vi "IMAQController.SaveImages.vi"(0 "Scan Variables":T1, 1 "Save path in":path, 2 "Scan running?":bool, 3 "Acquisition Mode":T2(ring), 4 "serviceName":string, 5 "error in (no error)":errorcluster) -> (14 "Save path out Scan folder":path, 15 "Save path out Rainbow":path, 16 "Save path out Original":path, 17 "Save path out Horizontal":path, 18 "Save path out Verical":path, 19 "error out":errorcluster)   [LabVIEW 2014, in "IMAQController.lvlib"]
uses:
  IMAQController.lvlib
  CSlibraries-extern/DimLVEvent/LVDimInterface/LVDimInterface.lvlib
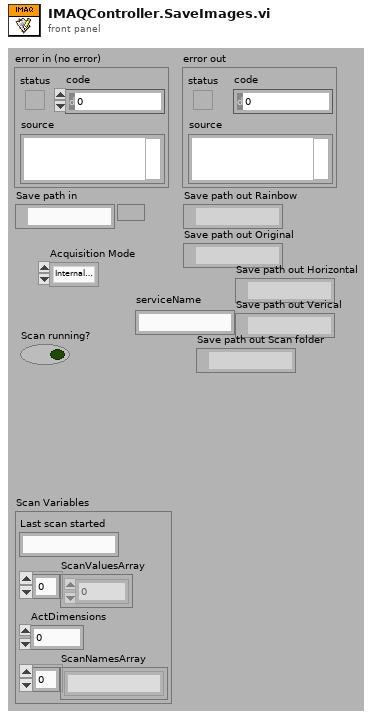
[diagram p1: front panel]
types:
  T1 = cluster{"Last scan started":string, "ScanValuesArray":dbl[], "ActDimensions":i16, "ScanNamesArray":string[]}
  T2 = enum32{"Internal Trigger", "Scan", "free Running", "External Trigger"}
  T3 = typedef "LVDateTimeRec.ctl" = cluster{"fractional second":dbl, "second":i32, "minute":i32, "hour":i32, "day of month":i32, "month":i32, "year":i32, "day of week":i32, "day of year":i32, "DST":i32}
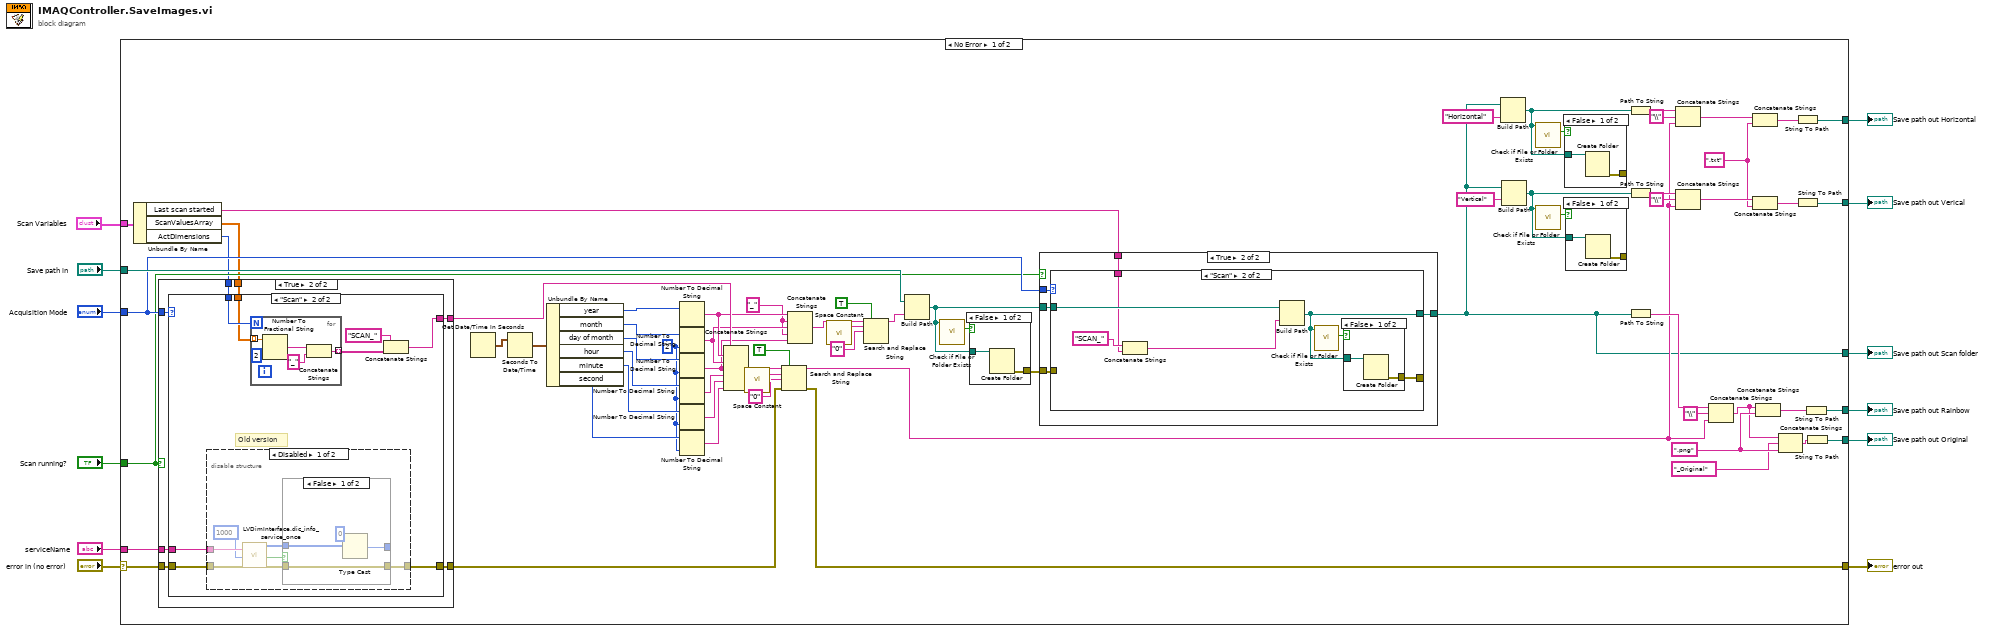
[diagram p0: block diagram]
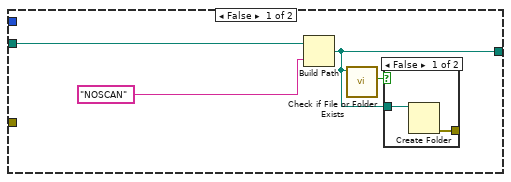
[diagram p2: hidden frame]
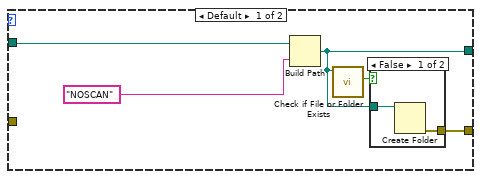
[diagram p4: hidden frame]
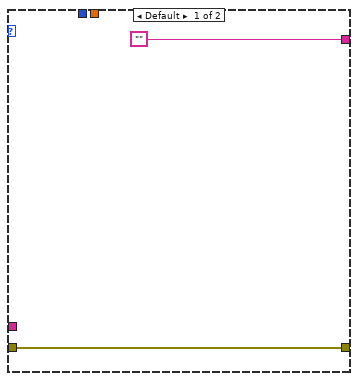
[diagram p8: hidden frame]
diagram:
  n1 = case shown="No Error" "error in (no error)" {
    selector: "error in (no error)" -> [w62 w150]
    tunnel: [w68 w150] -> w12
    tunnel: "Save path in" -> [w49 _]
    tunnel: [w64 _] -> w10
    tunnel: "Acquisition Mode" -> [w47 _]
    tunnel: "serviceName" -> [w60 _]
    tunnel: [w58 _] -> w7
    tunnel: [w21 _] -> w5
    tunnel: [w20 _] -> w4
    tunnel: "Scan Variables" -> [w19 _]
    tunnel: [w18 _] -> w3
    tunnel: "Scan running?" -> [w16 _]
    frame No Error {
      w24 = ".txt" ("string")
      w51 = "_"
      w56 = ".png" ("string")
      w70 = i16 2 ("width (-)")
      n2 = Unbundle By Name(w19) -> ("Last scan started"=w15:string, "ScanValuesArray"=w13:dbl[], "ActDimensions"=w14:i16)
      n3 = case shown="True" w16 {
        tunnel: [_ w115] -> w63
        tunnel: w62 -> [w108 w114]
        tunnel: [w108 w113] -> w61
        tunnel: w60 -> [_ w112]
        tunnel: w47 -> [_ w111]
        tunnel: w14 -> [_ w110]
        tunnel: w13 -> [_ w109]
        frame False {
        }
        frame True {
          n4 = case shown="\"Scan\"" w111 {
            tunnel: ["" w118] -> w115
            tunnel: w114 -> [w116 w125]
            tunnel: [w116 w123] -> w113
            tunnel: w112 -> [_ w124]
            tunnel: w110 -> [_ w122]
            tunnel: w109 -> [_ w121]
            frame Default {
            }
            frame "Scan" {
              # "Old version"
              n5 = disable-structure shown="Disabled" {
                disable-tunnel: w125 -> [w132 w138]
                disable-tunnel: w124 -> [w131 _]
                disable-tunnel: [w126 w138] -> w123
                frame Disabled {
                  n6 = call "LVDimInterface.dic_info_service_once.vi"("serviceName"=w131, "timeout [ms]"=u32 1000, "error in (no error)"=w132) -> ("data"=w129:i8[], "timed out?"=w127:bool, "error out"=w128:errorcluster)  [unwired: 13 in, 1 out]
                  n7 = case shown="False" w127 {
                    tunnel: w129 -> [w134 _]
                    tunnel: w128 -> [w133 w137]
                    tunnel: [w133 w137] -> w126
                    tunnel: [w136 _] -> _
                    frame False {
                      n8 = Type Cast(type=0, x=w134) -> (*(type *) &x=w136:i32)
                    }
                    frame True {
                    }
                  }
                }
                frame Enabled {
                }
              }
              n9 = for {
                N: w122 -> [_]
                tunnel: w121 -> [w143] mode=indexing
                tunnel: [w140] -> w120 mode=indexing
                n10 = Number To Fractional String(number=w143, precision (6)=i16 2) -> (F-format string=w142:string)  [unwired: 2 in]
                n11 = Concatenate Strings(w142, "_" ("string")) -> (w140:string)
              }
              n12 = Concatenate Strings("SCAN_", w120) -> (w118:string)
            }
          }
        }
      }
      n13 = Get Date/Time In Seconds() -> (seconds since 1Jan1904=w78:timestamp)
      n14 = Seconds To Date/Time(time stamp (now)=w78) -> (date time rec=w77:T3)  [unwired: 1 in]
      n15 = Unbundle By Name(w77) -> ("year"=w76:i32, "month"=w75:i32, "day of month"=w74:i32, "hour"=w73:i32, "minute"=w72:i32, "second"=w71:i32)
      n16 = Number To Decimal String(number=w76) -> (decimal integer string=w53:string)  [unwired: 1 in]
      n17 = Number To Decimal String(number=w75, width (-)=w70) -> (decimal integer string=w52:string)
      n18 = Number To Decimal String(number=w74, width (-)=w70) -> (decimal integer string=w50:string)
      n19 = Number To Decimal String(number=w73, width (-)=w70) -> (decimal integer string=w45:string)
      n20 = Number To Decimal String(number=w72, width (-)=w70) -> (decimal integer string=w44:string)
      n21 = Number To Decimal String(number=w71, width (-)=w70) -> (decimal integer string=w43:string)
      n22 = Concatenate Strings(w63, w53, w52, w50, w45, w44, w43) -> (w69:string)
      n23 = call <vilib>:"Space Constant.vi"() -> ("String"=w66:string)
      n24 = Search and Replace String(replace all?=TRUE ("replace all? (F)"), input string=w69, search string=w66, replace string="0" ("replace string (\"\")"), error in=w61) -> (result string=w27:string, error out=w68:errorcluster)  [unwired: 3 in, 2 out]
      n25 = Concatenate Strings(w53, w51, w52, w51, w50) -> (w39:string)
      n26 = call <vilib>:"Space Constant.vi"() -> ("String"=w41:string)
      n27 = Search and Replace String(replace all?=TRUE ("replace all? (F)"), input string=w39, search string=w41, replace string="0" ("replace string (\"\")")) -> (result string=w38:string)  [unwired: 4 in, 3 out]
      n28 = Build Path(base path=w49, name or relative path=w38) -> (appended path=w46:path)
      n29 = call <vilib>:"Check if File or Folder Exists.vi"("path"=w46) -> ("file or folder exists?"=w48:bool)  [unwired: 8 in, 2 out]
      n30 = case shown="False" w48 {
        tunnel: w46 -> [w149 _]
        tunnel: [w148 _] -> w17
        frame False {
          n31 = Create Folder(path (use dialog)=w149) -> (error out=w148:errorcluster)  [unwired: 2 in, 2 out]
        }
        frame True {
        }
      }
      n32 = case shown="True" w16 {
        tunnel: w47 -> [_ w91]
        tunnel: w46 -> [w82 w90]
        tunnel: w15 -> [_ w89]
        tunnel: [w81 w88] -> w18
        tunnel: w17 -> [_ w87]
        frame False {
          n33 = Build Path(base path=w82, name or relative path="NOSCAN" ("string")) -> (appended path=w81:path)
          n34 = call <vilib>:"Check if File or Folder Exists.vi"("path"=w81) -> ("file or folder exists?"=w84:bool)  [unwired: 8 in, 2 out]
          n35 = case shown="False" w84 {
            tunnel: w81 -> [w86 _]
            tunnel: [w85 _] -> _
            frame False {
              n36 = Create Folder(path (use dialog)=w86) -> (error out=w85:errorcluster)  [unwired: 2 in, 2 out]
            }
            frame True {
            }
          }
        }
        frame True {
          n37 = case shown="\"Scan\"" w91 {
            tunnel: w90 -> [w95 w104]
            tunnel: [w94 w102] -> w88
            tunnel: w89 -> [_ w100]
            tunnel: w87 -> [_ _]
            tunnel: [w92 w99] -> _
            frame Default {
              n38 = Build Path(base path=w95, name or relative path="NOSCAN" ("string")) -> (appended path=w94:path)
              n39 = call <vilib>:"Check if File or Folder Exists.vi"("path"=w94) -> ("file or folder exists?"=w96:bool)  [unwired: 8 in, 2 out]
              n40 = case shown="False" w96 {
                tunnel: w94 -> [w98 _]
                tunnel: [w97 _] -> w92
                frame False {
                  n41 = Create Folder(path (use dialog)=w98) -> (error out=w97:errorcluster)  [unwired: 2 in, 2 out]
                }
                frame True {
                }
              }
            }
            frame "Scan" {
              n42 = Concatenate Strings("SCAN_" ("string"), w100) -> (w101:string)
              n43 = Build Path(base path=w104, name or relative path=w101) -> (appended path=w102:path)
              n44 = call <vilib>:"Check if File or Folder Exists.vi"("path"=w102) -> ("file or folder exists?"=w105:bool)  [unwired: 8 in, 2 out]
              n45 = case shown="False" w105 {
                tunnel: w102 -> [w107 _]
                tunnel: [w106 _] -> w99
                frame False {
                  n46 = Create Folder(path (use dialog)=w107) -> (error out=w106:errorcluster)  [unwired: 2 in, 2 out]
                }
                frame True {
                }
              }
            }
          }
        }
      }
      n47 = Build Path(base path=w18, name or relative path="Horizontal") -> (appended path=w33:path)
      n48 = Build Path(base path=w18, name or relative path="Vertical") -> (appended path=w32:path)
      n49 = call <vilib>:"Check if File or Folder Exists.vi"("path"=w33) -> ("file or folder exists?"=w37:bool)  [unwired: 8 in, 2 out]
      n50 = call <vilib>:"Check if File or Folder Exists.vi"("path"=w32) -> ("file or folder exists?"=w36:bool)  [unwired: 8 in, 2 out]
      n51 = case shown="False" w37 {
        tunnel: w33 -> [w147 _]
        tunnel: [w146 _] -> _
        frame False {
          n52 = Create Folder(path (use dialog)=w147) -> (error out=w146:errorcluster)  [unwired: 2 in, 2 out]
        }
        frame True {
        }
      }
      n53 = case shown="False" w36 {
        tunnel: w32 -> [w145 _]
        tunnel: [w144 _] -> _
        frame False {
          n54 = Create Folder(path (use dialog)=w145) -> (error out=w144:errorcluster)  [unwired: 2 in, 2 out]
        }
        frame True {
        }
      }
      n55 = Path To String(path=w33) -> (string=w30:string)
      n56 = Path To String(path=w32) -> (string=w28:string)
      n57 = Path To String(path=w18) -> (string=w80:string)
      n58 = Concatenate Strings(w30, "\\" ("string"), w27) -> (w26:string)
      n59 = Concatenate Strings(w28, "\\" ("string"), w27) -> (w25:string)
      n60 = Concatenate Strings(w80, "\\" ("string"), w27) -> (w54:string)
      n61 = Concatenate Strings(w26, w24) -> (w23:string)
      n62 = Concatenate Strings(w25, w24) -> (w22:string)
      n63 = Concatenate Strings(w54, w56) -> (w57:string)
      n64 = Concatenate Strings(w54, "_Original" ("string"), w56) -> (w59:string)
      n65 = String To Path(string=w23) -> (path=w21:path)
      n66 = String To Path(string=w22) -> (path=w20:path)
      n67 = String To Path(string=w57) -> (path=w64:path)
      n68 = String To Path(string=w59) -> (path=w58:path)
    }
    frame Error {
    }
  }
  "error out" <- w12
  "Save path out Rainbow" <- w10
  "Save path out Original" <- w7
  "Save path out Horizontal" <- w5
  "Save path out Verical" <- w4
  "Save path out Scan folder" <- w3
